vi "Get Channel Name.vi"(8 "error in (no error)":errorcluster, 10 "index":i32, 11 "Impulse Manager in":refnum<class "Impulse Manager.lvclass">) -> (0 "error out":errorcluster, 2 "Channel Name":string, 3 "Impulse Manager out":refnum<class "Impulse Manager.lvclass">)   [LabVIEW 2016, in "Impulse Manager.lvclass"]
uses:
  Impulse Manager.lvclass
  Impulse Manager.lvclass/Impulse Manager.ctl
  Impulse Data/Impulse Data.lvclass
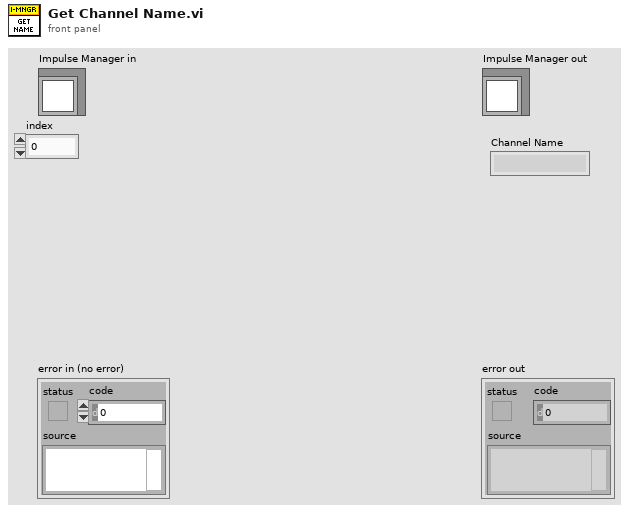
[diagram p1: front panel]
types:
  T1 = typedef "Impulse Data.lvclass/Instance handle.ctl" = refnum<data-value>
  T2 = typedef "core.lvlib/TD_Impulse Parameter.ctl" = cluster{"Color":u32, "Visible":bool, "Channel":u16, "Invert":bool, "Desaccade":bool, "Offset":dbl, "Gain":dbl}[]
  T3 = cluster{"Color":u32, "Visible":bool, "Channel":u16, "Invert":bool, "Desaccade":bool, "Offset":dbl, "Gain":dbl}
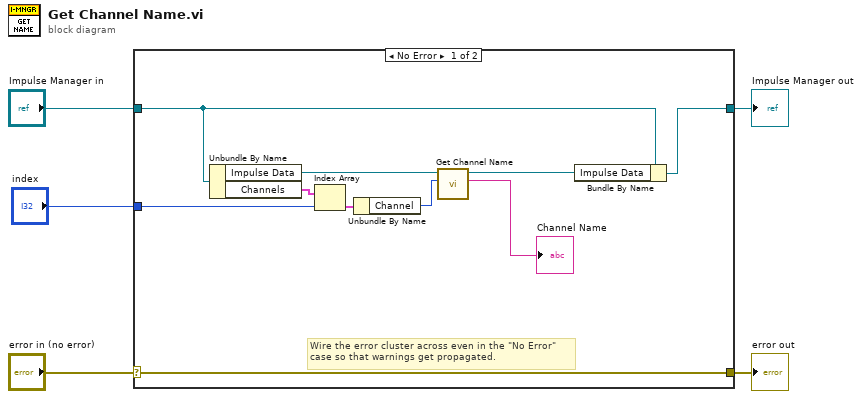
[diagram p0: block diagram]
diagram:
  n1 = case shown="No Error" "error in (no error)" {
    selector: "error in (no error)" -> [w15 w17]
    tunnel: [w15 w17] -> w4
    tunnel: [w6 w16] -> w2
    tunnel: "Impulse Manager in" -> [w7 w16]
    tunnel: "index" -> [w13 _]
    frame No Error {
      # "Wire the error cluster across even in the \"No Error\"\ncase so that warnings get propagated."
      n2 = Unbundle By Name(w7) -> ("Impulse Data"=w11:T1, "Channels"=w14:T2)
      n3 = Index Array(array=w14, index=w13) -> (element=w12:T3)
      n4 = Unbundle By Name(w12) -> ("Channel"=w10:u16)
      n5 = call "Get Channel Name.vi"("index"=w10, "Impulse Data in"=w11) -> ("Channel Name"=→"Channel Name":string, "Impulse Data out"=w8:T1)  [unwired: 7 in, 1 out]
      n6 = Bundle By Name(cluster=w7, "Impulse Data"=w8) -> (w6:refnum<class "Impulse Manager.lvclass">)
    }
    frame Error {
    }
  }
  "error out" <- w4
  "Impulse Manager out" <- w2
